vi "Log_logtofile.vi"(6 "Waveform Chart in":dbl, 7 "y":dbl, 9 "Temperature setpoint":dbl, 10 "Start_stop_file_writing":bool, 11 "Data file name:":path) -> ()   [LabVIEW 2018]
uses:
  <vilib>/Utility/file.llb/Write Delimited Spreadsheet (string).vi
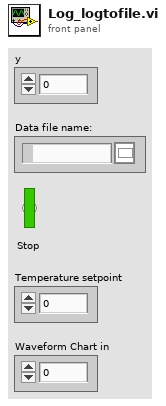
[diagram p1: front panel]
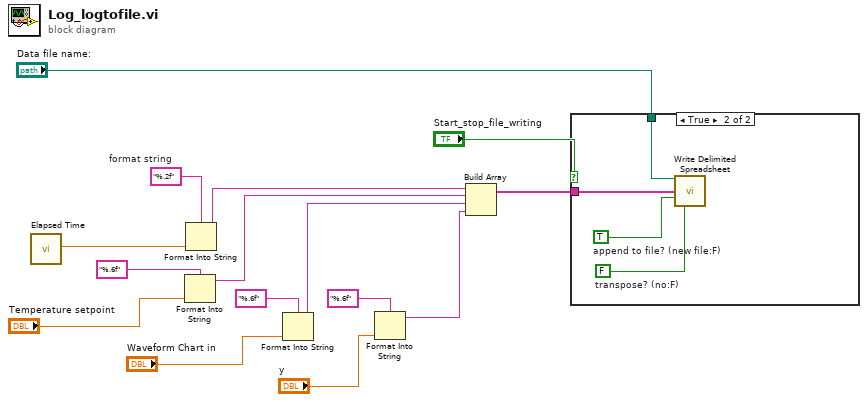
[diagram p0: block diagram]
diagram:
  w1 = "%.2f"  # format string
  n1 = call "Elapsed Time"() -> ("Elapsed Time (s)"=w5:dbl)  [unwired: 12 in, 7 out]
  n2 = Format Into String(format string="%.6f", "Temperature setpoint") -> (resulting string=w3:string)  [unwired: 2 in, 1 out]
  n3 = Format Into String "Format Into String"(format string=w1, w5) -> (resulting string=w2:string)  [unwired: 2 in, 1 out]
  n4 = Format Into String(format string="%.6f", "Waveform Chart in") -> (resulting string=w9:string)  [unwired: 2 in, 1 out]
  n5 = Format Into String(format string="%.6f", "y") -> (resulting string=w13:string)  [unwired: 2 in, 1 out]
  n6 = Build Array "Build Array"(w2, w3, w9, w13) -> (w6:string[])
  n7 = case shown="True" "Start_stop_file_writing" {
    tunnel: w6 -> [_ w17]
    tunnel: "Data file name:" -> [_ w16]
    frame False {
    }
    frame True {
      w19 = TRUE  # append to file? (new file:F)
      w18 = FALSE  # transpose? (no:F)
      n8 = call-poly <vilib>:"Write Delimited Spreadsheet.vi"("file path (dialog if empty)"=w16, "1D data"=w17, "append to file? (new file:F)"=w19, "transpose? (no:F)"=w18) -> ()  [unwired: 10 in, 2 out]
    }
  }
